vi "Disabled.vi"(7 "Robot Mode":T17, 8 "Driver Command_Inputs":T1, 9 "Sensor Inputs (in)":T9, 10 "Match Info":T16={"Autonomous Elapsed Seconds"=0.0, "TeleOp Elapsed Seconds"=0.0, "Disabled Elapsed Seconds"=0.0, "Visited Autonomous"=FALSE, "Visited TeleOp"=FALSE, "Visited Disabled"=FALSE, "Autonomous Settings"={"Autonomous Style"=enum."Independent", "VI Refnum"=refnum}}, 11 "Call Context":T18) -> (2 "Disabled Commands":T1, 3 "Sensor Inputs (out)":T9)   [LabVIEW 2012]
doc: "This VI is called each time a disabled packet is received from the DS. It is often used to prepare for the next robot mode, to calibrate sensors, etc."
uses:
  <vilib>/Rock Robotics/WPI/DriverStation/WPI_DriverStationDerivedRobotMode.ctl
  <vilib>/Rock Robotics/WPI/DriverStation/WPI_DriverStationRobotMode.ctl
  <vilib>/Rock Robotics/WPI/DriverStation/WPI_DriverStationMatch Info.ctl
  Inputs_All.ctl
  Flywheel/Sensor_Inputs_FlyWheel.ctl
  tankdrive/Input_Sensors_Drive.ctl
  Conveyor/Sensor_Input_Conveyor.ctl
  Conveyor/Sensor_Input_ConveyorV2.ctl
  Turret/Inputs_Sensors_Turret.ctl
  Inputs_Camera.ctl
  Command_Inputs.ctl
  tankdrive/Input_Commands_Drive.ctl
  Conveyor/Input_Command_Conveyor.ctl
  Turret/Inputs_Commands_Turret.ctl
  Bridge Tipper/Inputs_Tipper.ctl
  Dashboard Controls.ctl
  Roller/Input_Commands_Roller.ctl
  Flywheel/Input_Commands_Flywheel.ctl
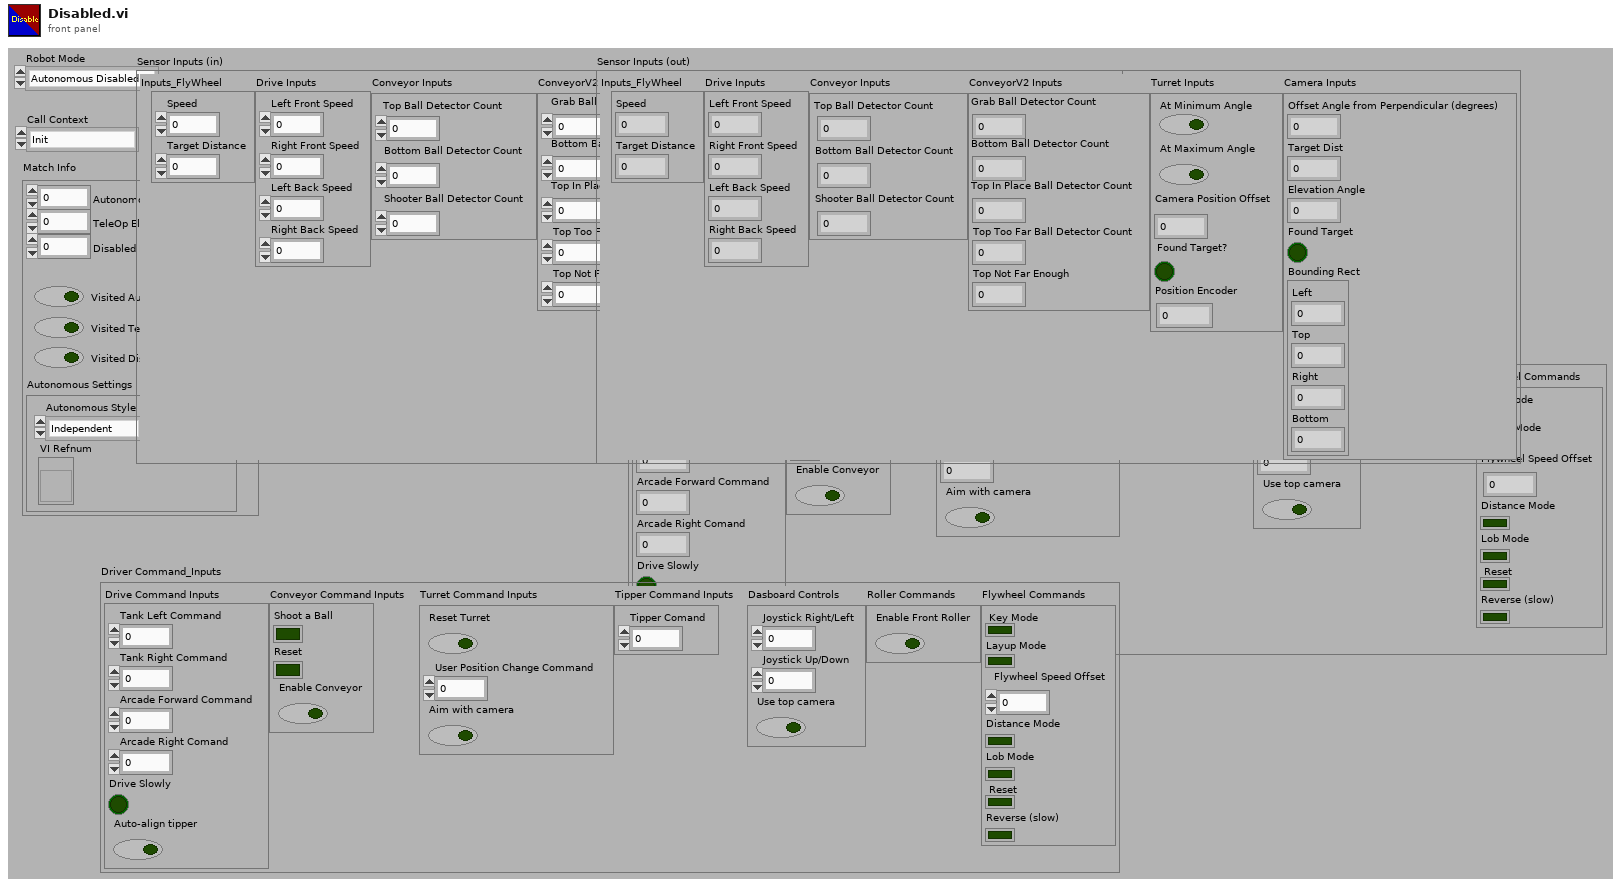
[diagram p1: front panel]
types:
  T1 = typedef "Command_Inputs.ctl" = cluster{"Drive Command Inputs":T2, "Conveyor Command Inputs":T3, "Turret Command Inputs":T4, "Tipper Command Inputs":T5, "Dasboard Controls":T6, "Roller Commands":T7, "Flywheel Commands":T8}
  T2 = typedef "Input_Commands_Drive.ctl" = cluster{"Tank Left Command":dbl, "Tank Right Command":dbl, "Arcade Forward Command":dbl, "Arcade Right Comand":dbl, "Drive Slowly":bool, "Auto-align tipper":bool}
  T3 = typedef "Input_Command_Conveyor.ctl" = cluster{"Shoot a Ball":bool, "Reset":bool, "Enable Conveyor":bool}
  T4 = typedef "Inputs_Commands_Turret.ctl" = cluster{"Reset Turret":bool, "User Position Change Command":dbl, "Aim with camera":bool}
  T5 = typedef "Inputs_Tipper.ctl" = cluster{"Tipper Comand":dbl}
  T6 = typedef "Dashboard Controls.ctl" = cluster{"Joystick Right/Left":dbl, "Joystick Up/Down":dbl, "Use top camera":bool}
  T7 = typedef "Input_Commands_Roller.ctl" = cluster{"Enable Front Roller":bool}
  T8 = typedef "Input_Commands_Flywheel.ctl" = cluster{"Key Mode":bool, "Layup Mode":bool, "Flywheel Speed Offset":dbl, "Distance Mode":bool, "Lob Mode":bool, "Reset":bool, "Reverse (slow)":bool}
  T9 = typedef "Inputs_All.ctl" = cluster{"Inputs_FlyWheel":T10, "Drive Inputs":T11, "Conveyor Inputs":T12, "ConveyorV2 Inputs":T13, "Turret Inputs":T14, "Camera Inputs":T15}
  T10 = typedef "Sensor_Inputs_FlyWheel.ctl" = cluster{"Speed":dbl, "Target Distance":dbl}
  T11 = typedef "Input_Sensors_Drive.ctl" = cluster{"Left Front Speed":dbl, "Right Front Speed":dbl, "Left Back Speed":dbl, "Right Back Speed":dbl}
  T12 = typedef "Sensor_Input_Conveyor.ctl" = cluster{"Top Ball Detector Count":i32, "Bottom Ball Detector Count":i32, "Shooter Ball Detector Count":i32}
  T13 = typedef "Sensor_Input_ConveyorV2.ctl" = cluster{"Grab Ball Detector Count":i32, "Bottom Ball Detector Count":i32, "Top In Place Ball Detector Count":i32, "Top Too Far Ball Detector Count":i32, "Top Not Far Enough":i32}
  T14 = typedef "Inputs_Sensors_Turret.ctl" = cluster{"At Minimum Angle":bool, "At Maximum Angle":bool, "Camera Position Offset":dbl, "Found Target?":bool, "Position Encoder":dbl}
  T15 = typedef "Inputs_Camera.ctl" = cluster{"Offset Angle from Perpendicular (degrees)":dbl, "Target Dist":dbl, "Elevation Angle":dbl, "Found Target":bool, "Bounding Rect":cluster{"Left":dbl, "Top":dbl, "Right":dbl, "Bottom":dbl}}
  T16 = typedef "WPI_DriverStationMatch Info.ctl" = cluster{"Autonomous Elapsed Seconds":dbl, "TeleOp Elapsed Seconds":dbl, "Disabled Elapsed Seconds":dbl, "Visited Autonomous":bool, "Visited TeleOp":bool, "Visited Disabled":bool, "Autonomous Settings":cluster{"Autonomous Style":enum16{"Iterative", "Independent"}, "VI Refnum":refnum<vi>}}
  T17 = typedef "WPI_DriverStationRobotMode.ctl" = enum16{"Autonomous Disabled", "Autonomous Enabled", "Teleop Disabled", "Teleop Enabled", "Timeout", "Finish"}
  T18 = typedef "WPI_DriverStationDerivedRobotMode.ctl" = enum16{"Init", "Execute", "Stop"}
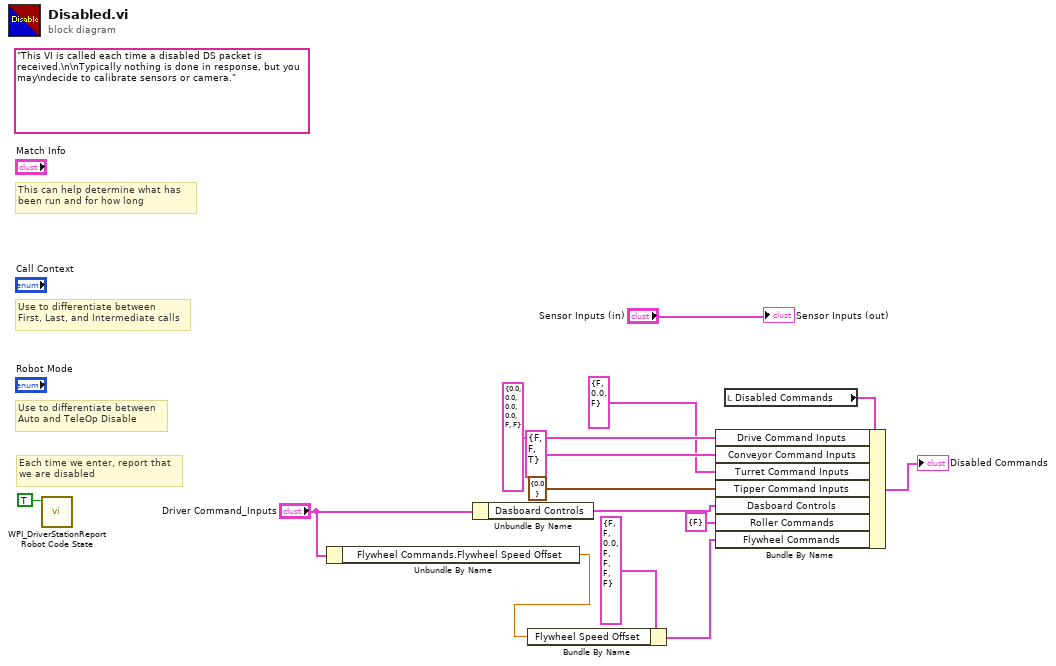
[diagram p0: block diagram]
diagram:
  (unwired) "This VI is called each time a disabled DS packet is received.\n\nTypically nothing is done in response, but you may\ndecide to calibrate sensors or camera."
  # "Each time we enter, report that\nwe are disabled"
  # "Use to differentiate between\nFirst, Last, and Intermediate calls"
  # "This can help determine what has\nbeen run and for how long"
  # "Use to differentiate between\nAuto and TeleOp Disable"
  n1 = call <vilib>:"WPI_DriverStationReport Robot Code State.vi"("Disabled"=TRUE ("Autonomous")) -> ()  [unwired: 10 in, 1 out]
  n2 = Unbundle By Name("Driver Command_Inputs") -> ("Flywheel Commands.Flywheel Speed Offset"=w1:dbl)
  n3 = Unbundle By Name("Driver Command_Inputs") -> ("Dasboard Controls"=w6:T6)
  n4 = Bundle By Name(cluster=T8 {"Key Mode"=FALSE, "Layup Mode"=FALSE, "Flywheel Speed Offset"=0.0, "Distance Mode"=FALSE, "Lob Mode"=FALSE, "Reset"=FALSE, "Reverse (slow)"=FALSE} ("Flywheel Commands"), "Flywheel Speed Offset"=w1) -> (w2:T8)
  n5 = local read "Disabled Commands"() -> (w8:T1)
  n6 = Bundle By Name(cluster=w8, "Drive Command Inputs"=T2 {"Tank Left Command"=0.0, "Tank Right Command"=0.0, "Arcade Forward Command"=0.0, "Arcade Right Comand"=0.0, "Drive Slowly"=FALSE, "Auto-align tipper"=FALSE}, "Conveyor Command Inputs"=T3 {"Shoot a Ball"=FALSE, "Reset"=FALSE, "Enable Conveyor"=TRUE}, "Turret Command Inputs"=T4 {"Reset Turret"=FALSE, "User Position Change Command"=0.0, "Aim with camera"=FALSE}, "Tipper Command Inputs"=T5 {"Tipper Comand"=0.0}, "Dasboard Controls"=w6, "Roller Commands"=T7 {"Enable Front Roller"=FALSE}, "Flywheel Commands"=w2) -> (→"Disabled Commands":T1)
  "Sensor Inputs (out)" <- "Sensor Inputs (in)"
